vi "Cleanup.vi"(8 "error in (no error)":errorcluster, 11 "VisaComms in":refnum<class "VisaComms.lvclass">) -> (0 "error out":errorcluster)   [LabVIEW 2020, in "CTI.lvlib" / "VisaComms.lvclass"]
uses:
  VisaComms.lvclass
  VisaComms.lvclass/VisaComms.ctl
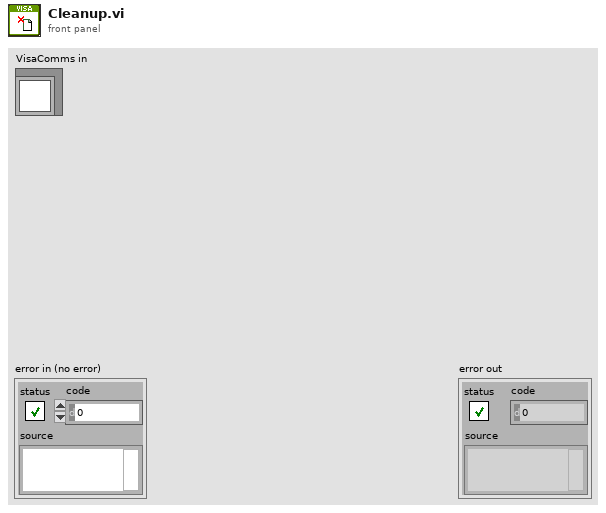
[diagram p1: front panel]
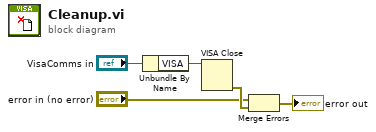
[diagram p0: block diagram]
diagram:
  n1 = Unbundle By Name("VisaComms in") -> ("VISA"=w4:refnum<visa-resource-name>)
  n2 = VISA Close(VISA resource name=w4) -> (error out=w3:errorcluster)  [unwired: 1 in]
  n3 = Merge Errors("error in (no error)", w3) -> (→"error out":errorcluster)
